vi "To String (Boolean).vi"(0 "Variant in":variant, 11 "error in (no error)":errorcluster) -> (4 "String":string, 15 "error out":errorcluster)   [LabVIEW 2017, in "Variant JSON API.lvlib"]
uses:
  Variant JSON API.lvlib
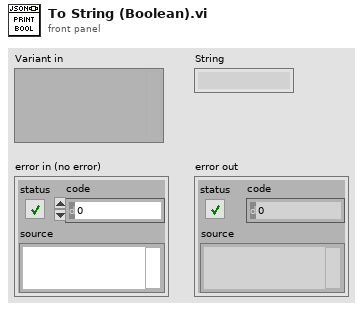
[diagram p1: front panel]
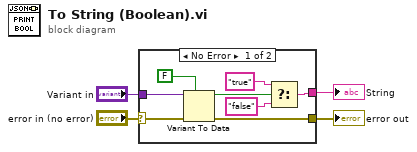
[diagram p0: block diagram]
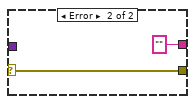
[diagram p2: hidden frame]
diagram:
  n1 = case shown="No Error" "error in (no error)" {
    selector: "error in (no error)" -> [w7 w13]
    tunnel: "Variant in" -> [w12 _]
    tunnel: [w9 "" ("f")] -> w3
    tunnel: [w6 w13] -> w1
    frame No Error {
      n2 = Variant To Data(error in=w7, type=FALSE, Variant=w12) -> (data=w5:bool, error out=w6:errorcluster)
      n3 = Select(t="true" ("String"), s=w5, f="false") -> (s? t:f=w9:string)
    }
    frame Error {
    }
  }
  "String" <- w3
  "error out" <- w1
